vi "74HC112设计2-4分频器.vi"() -> ()   [LabVIEW 2018]
panel:
  in  "结束":bool
  out "Q2":bool
  out "Q1":bool
  in  "cp":bool
  # "74HC112：JK触发器"
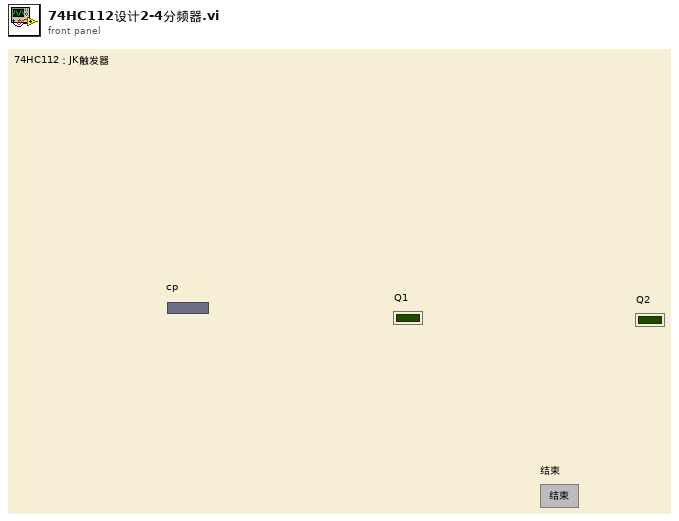
[diagram p1: front panel]
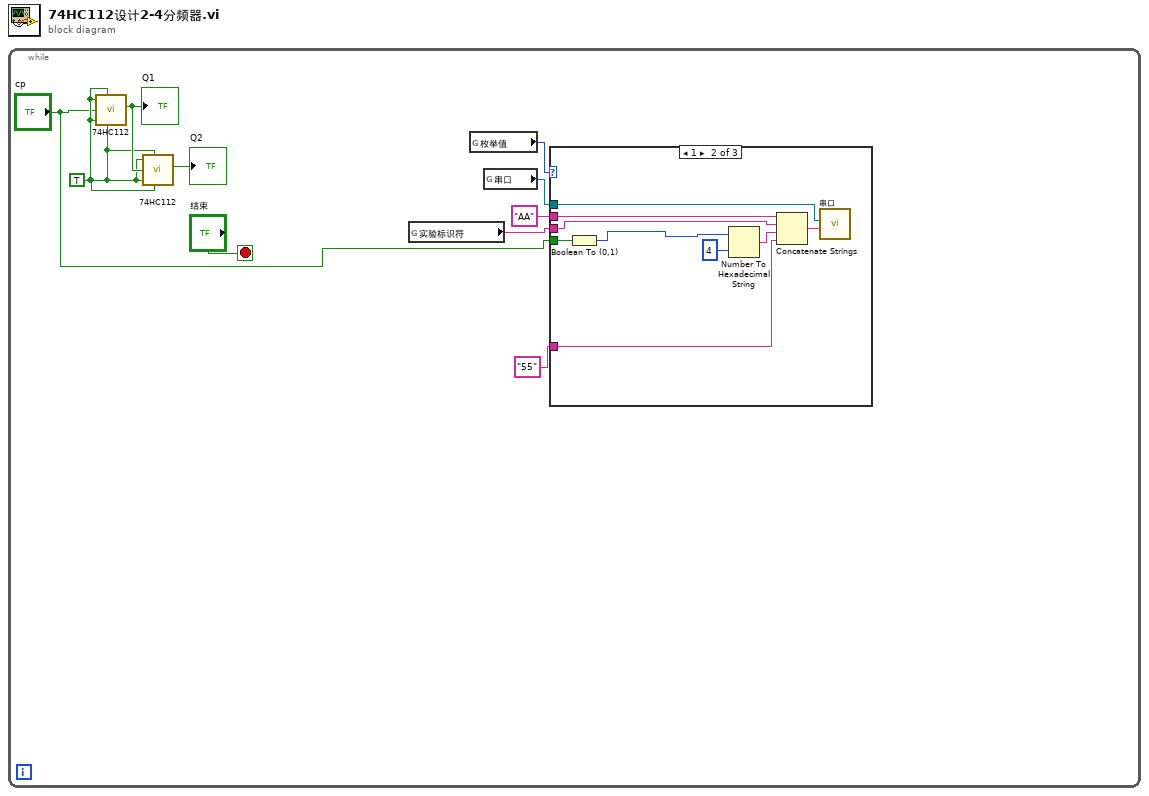
[diagram p0: block diagram]
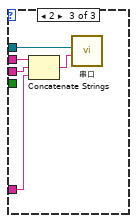
[diagram p3: hidden frame]
diagram:
  n1 = while {
    stop <- "结束" stop-if-true
    w8 = TRUE
    n2 = call "74HC112.vi"("J"=w8, "R"=w8, "cp"="cp", "K"=w8, "S"=w8) -> ("Q"=w10:bool)  [unwired: 2 in, 1 out]
    "Q1" <- w10
    n3 = call "74HC112.vi"("J"=w8, "R"=w8, "cp"=w10, "K"=w8, "S"=w8) -> ("Q"=→"Q2":bool)  [unwired: 2 in, 1 out]
    n4 = global read "全局变量.vi" "实验标识符"() -> (w4:string)
    n5 = global read "全局变量.vi" "枚举值"() -> (w6:i8)
    n6 = global read "全局变量.vi" "串口"() -> (w5:refnum<visa-resource-name>)
    n7 = case shown="1" w6 {
      tunnel: "cp" -> [_ w18 _]
      tunnel: w5 -> [_ w17 w22]
      tunnel: w4 -> [_ w16 w23]
      tunnel: "55" -> [_ w15 w20]
      tunnel: "AA" -> [_ w14 w21]
      frame 0, Default {
      }
      frame 1 {
        n8 = Boolean To (0,1)(Boolean=w18) -> (0, 1=w11:i16)
        n9 = Number To Hexadecimal String(1:4, 2:w11) -> (0:w12:string)
        n10 = Concatenate Strings(w14, w16, w12, w15) -> (w19:string)
        n11 = call "串口.vi"("字符串"=w19, "VISA resource name"=w17) -> ()  [unwired: 10 in]
      }
      frame 2 {
        n12 = Concatenate Strings(w21, w23, w20) -> (w24:string)
        n13 = call "串口.vi"("字符串"=w24, "VISA resource name"=w22) -> ()  [unwired: 10 in]
      }
    }
  }
